vi "GEA2 Register for Multiple Events.vi"(0 "GEA2 Reference Array In":refnum<k24>[](array[refnum]), 11 "Error In":errorcluster) -> (4 "GEA2 Reference Array Out":refnum<k24>[](array[refnum]), 8 "GEA2 Event Registration":refnum<event-registration>, 15 "Error Out":errorcluster)   [LabVIEW 2014, in "GEA2_Toolkit.lvlib"]
doc: "This VI registers for multiple events such that any messages that appear on multiple GEA2 buses will trigger events in LabVIEW. This event can be wired into an event structure and all messages received can be handled."
uses:
  library/GEA2_Toolkit.lvlib
  C:/Automation/DLLs/Appliance .NET/GeaCommunication.dll
  type defs/Data Out.ctl
  GEA2 Message Event Handler.vi
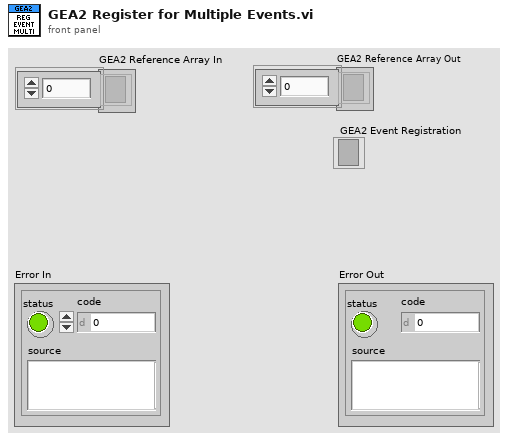
[diagram p1: front panel]
types:
  T1 = typedef "GEA2_Toolkit.lvlib/Data Out.ctl" = cluster{"Source":u8, "Destination":u8, "Command":u8, "Length":u8, "CRC":u16, "Message":string}
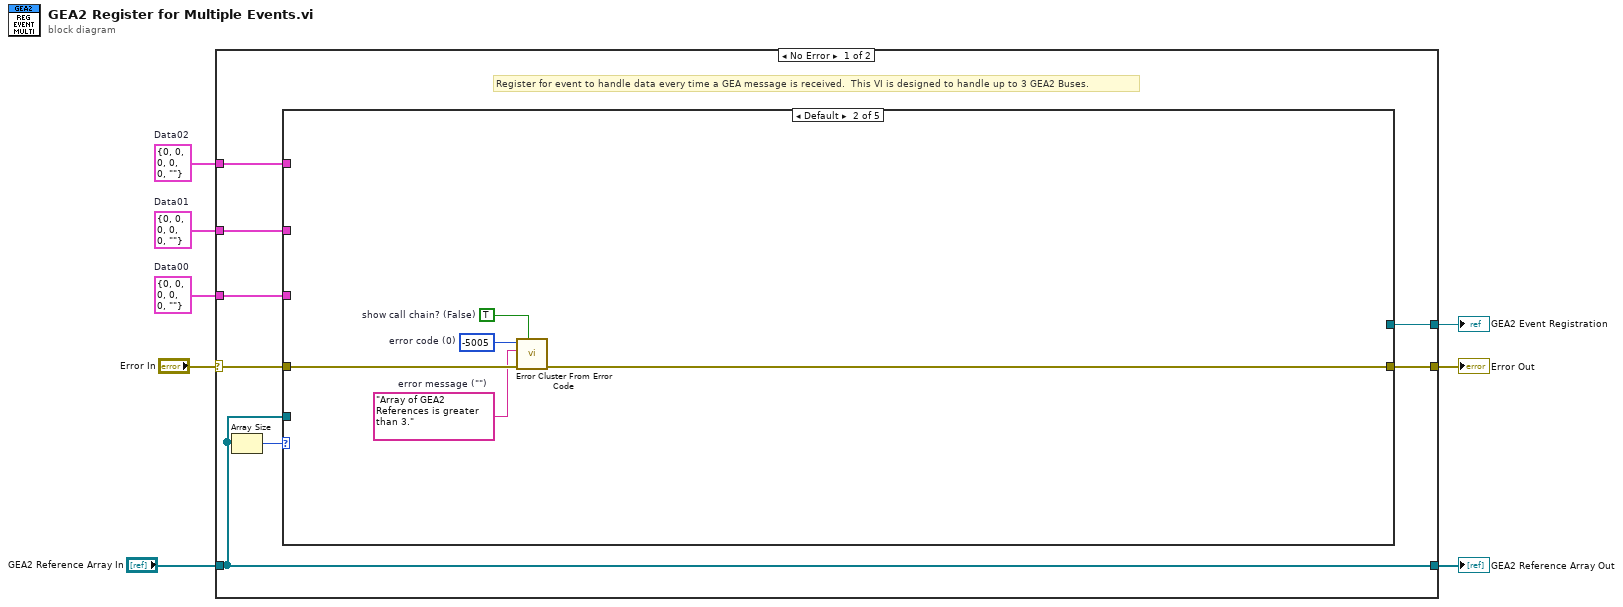
[diagram p0: block diagram]
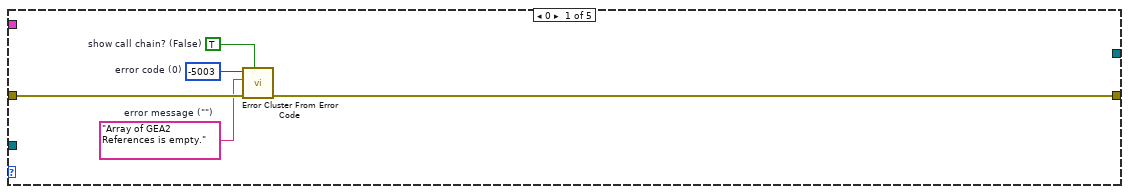
[diagram p2: hidden frame]
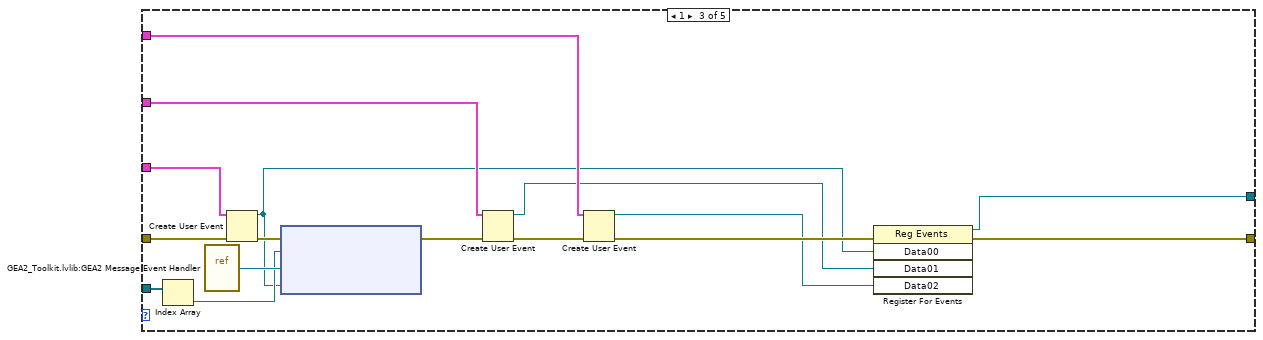
[diagram p3: hidden frame]
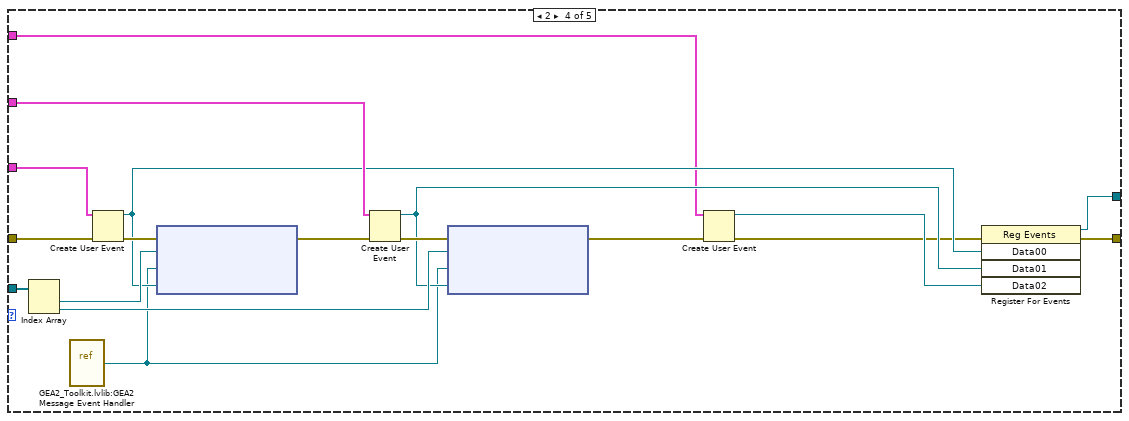
[diagram p4: hidden frame]
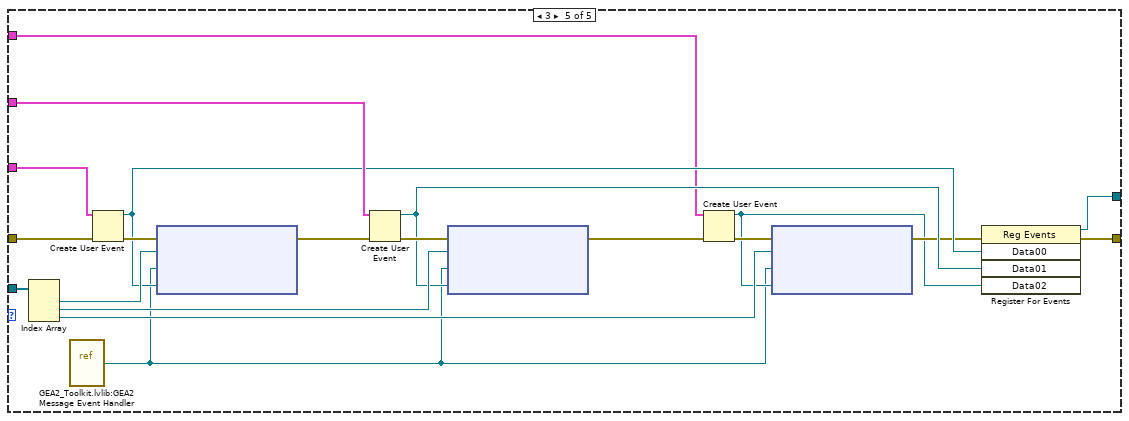
[diagram p5: hidden frame]
diagram:
  w3 = T1 {"Source"=0, "Destination"=0, "Command"=0, "Length"=0, "CRC"=0, "Message"=""}  # Data02
  w4 = T1 {"Source"=0, "Destination"=0, "Command"=0, "Length"=0, "CRC"=0, "Message"=""}  # Data01
  w1 = T1 {"Source"=0, "Destination"=0, "Command"=0, "Length"=0, "CRC"=0, "Message"=""}  # Data00
  n1 = case shown="No Error" "Error In" {
    selector: "Error In" -> [w15 w82]
    tunnel: [w16 w82] -> w8
    tunnel: "GEA2 Reference Array In" -> [w14 w81]
    tunnel: [w14 w81] -> w5
    tunnel: w4 -> [w13 _]
    tunnel: w3 -> [w12 _]
    tunnel: [w11 _] -> w2
    tunnel: w1 -> [w10 _]
    frame No Error {
      # "Register for event to handle data every time a GEA message is received.  This VI is designed to handle up to 3 GEA2 Buses."
      n2 = Array Size(array=w14) -> (size(s)=w9:i32)
      n3 = case shown="Default" w9 {
        tunnel: [w17 w22 w42 w60 w80] -> w16
        tunnel: w15 -> [w21 w26 w41 w59 w79]
        tunnel: w14 -> [_ _ w38 w57 w77]
        tunnel: w10 -> [_ _ w31 w55 w75]
        tunnel: w13 -> [_ _ w32 w53 w73]
        tunnel: w12 -> [_ _ w33 w48 w68]
        tunnel: [_ _ w27 w44 w62] -> w11
        frame 0 {
          w18 = TRUE  # show call chain? (False)
          w19 = "Array of GEA2 References is empty."  # error message ("")
          w20 = -5003  # error code (0)
          n4 = call <vilib>:"Error Cluster From Error Code.vi"("show call chain? (False)"=w18, "error in (no error)"=w21, "error message (\"\")"=w19, "error code (0)"=w20) -> ("error out"=w17:errorcluster)  [unwired: 5 in]
        }
        frame Default {
          w23 = TRUE  # show call chain? (False)
          w24 = "Array of GEA2 References is greater than 3."  # error message ("")
          w25 = -5005  # error code (0)
          n5 = call <vilib>:"Error Cluster From Error Code.vi"("show call chain? (False)"=w23, "error in (no error)"=w26, "error message (\"\")"=w24, "error code (0)"=w25) -> ("error out"=w22:errorcluster)  [unwired: 5 in]
        }
        frame 1 {
          n6 = Index Array(array=w38) -> (element=w37:refnum<k24>)  [unwired: 1 in]
          n7 = vi-ref "GEA2_Toolkit.lvlib:GEA2 Message Event Handler.vi"() -> (w39:refnum<vi>)
          n8 = Create User Event(user event datatype=w31, error in=w41) -> (user event=w30:refnum<user-event>, error out=w40:errorcluster)
          n9 = node(w40, w37, w39, w30) -> (w36:errorcluster)  [unwired: 1 in, 1 out]
          n10 = Create User Event(user event datatype=w32, error in=w36) -> (user event=w28:refnum<user-event>, error out=w35:errorcluster)
          n11 = Create User Event(user event datatype=w33, error in=w35) -> (user event=w29:refnum<user-event>, error out=w34:errorcluster)
          n12 = register-events(error in=w34, w30, w28, w29) -> (reference out=w27:refnum<event-registration>, error out=w42:errorcluster)  [unwired: 1 in]
        }
        frame 2 {
          n13 = Index Array(array=w57) -> (element #1=w56:refnum<k24>, element #2=w51:refnum<k24>)  [unwired: 2 in]
          n14 = vi-ref "GEA2_Toolkit.lvlib:GEA2 Message Event Handler.vi"() -> (w43:refnum<vi>)
          n15 = Create User Event(user event datatype=w55, error in=w59) -> (user event=w50:refnum<user-event>, error out=w58:errorcluster)
          n16 = node(w58, w56, w43, w50) -> (w54:errorcluster)  [unwired: 1 in, 1 out]
          n17 = Create User Event(user event datatype=w53, error in=w54) -> (user event=w49:refnum<user-event>, error out=w52:errorcluster)
          n18 = node(w52, w51, w43, w49) -> (w47:errorcluster)  [unwired: 1 in, 1 out]
          n19 = Create User Event(user event datatype=w48, error in=w47) -> (user event=w46:refnum<user-event>, error out=w45:errorcluster)
          n20 = register-events(error in=w45, w50, w49, w46) -> (reference out=w44:refnum<event-registration>, error out=w60:errorcluster)  [unwired: 1 in]
        }
        frame 3 {
          n21 = Index Array(array=w77) -> (element #1=w76:refnum<k24>, element #2=w71:refnum<k24>, element #3=w65:refnum<k24>)  [unwired: 3 in]
          n22 = vi-ref "GEA2_Toolkit.lvlib:GEA2 Message Event Handler.vi"() -> (w61:refnum<vi>)
          n23 = Create User Event(user event datatype=w75, error in=w79) -> (user event=w70:refnum<user-event>, error out=w78:errorcluster)
          n24 = node(w78, w76, w61, w70) -> (w74:errorcluster)  [unwired: 1 in, 1 out]
          n25 = Create User Event(user event datatype=w73, error in=w74) -> (user event=w69:refnum<user-event>, error out=w72:errorcluster)
          n26 = node(w72, w71, w61, w69) -> (w67:errorcluster)  [unwired: 1 in, 1 out]
          n27 = Create User Event(user event datatype=w68, error in=w67) -> (user event=w63:refnum<user-event>, error out=w66:errorcluster)
          n28 = node(w66, w65, w61, w63) -> (w64:errorcluster)  [unwired: 1 in, 1 out]
          n29 = register-events(error in=w64, w70, w69, w63) -> (reference out=w62:refnum<event-registration>, error out=w80:errorcluster)  [unwired: 1 in]
        }
      }
    }
    frame Error {
    }
  }
  "Error Out" <- w8
  "GEA2 Reference Array Out" <- w5
  "GEA2 Event Registration" <- w2
